vi "GetNeoParams.vi"(4 "error in (no error)":errorcluster, 7 "Handle":i32) -> (0 "error out":errorcluster, 3 "cluster":cluster{"AOIHeight":i64, "AOIWidth":i64})   [LabVIEW 2014]
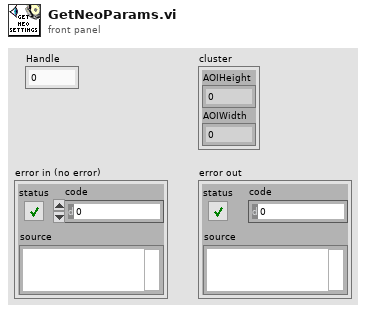
[diagram p1: front panel]
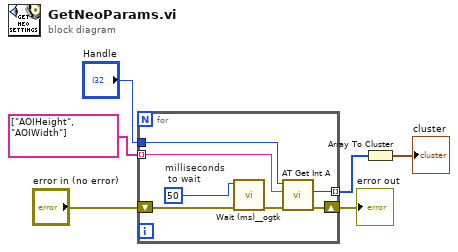
[diagram p0: block diagram]
diagram:
  n1 = for {
    tunnel: "Handle" -> [w13]
    shift-right: [w12] -> w6
    shift-left: "error in (no error)" -> [w9]
    tunnel: string[] ["AOIHeight", "AOIWidth"] -> [w11] mode=indexing
    tunnel: [w10] -> w3 mode=indexing
    w7 = u32 50  # milliseconds  to wait
    n2 = call <userlib>:"Wait (ms)__ogtk.vi"("error in (no error)"=w9, "milliseconds to wait"=w7) -> ("error out"=w8:errorcluster)  [unwired: 8 in, 1 out]
    n3 = call <userlib>:"AT Get Int A.vi"("error in (no error)"=w8, "Feature"=w11, "Handle"=w13) -> ("error out"=w12:errorcluster, "Value"=w10:i64)  [unwired: 6 in, 1 out]
  }
  "error out" <- w6
  n4 = Array To Cluster(array=w3) -> (cluster=→"cluster":cluster{"[0]":i64, "[1]":i64})
